vi "MQTT_TCP_Write.vi"(8 "error in (no error)":errorcluster, 9 "timeout ms (5000)":i32=5000, 10 "data in":u8[](array[numeric]) format="%x", 11 "connection ID":refnum<k5>) -> (0 "error out":errorcluster, 2 "bytes written":i32, 3 "connection ID out":refnum<k5>)   [LabVIEW 2012, in "MQTT_Functions.lvlib"]
uses:
  MQTT_Functions.lvlib
panel:
  # "this is just a wrapper for the TCP Write function\nadd or replace functionality as desired"
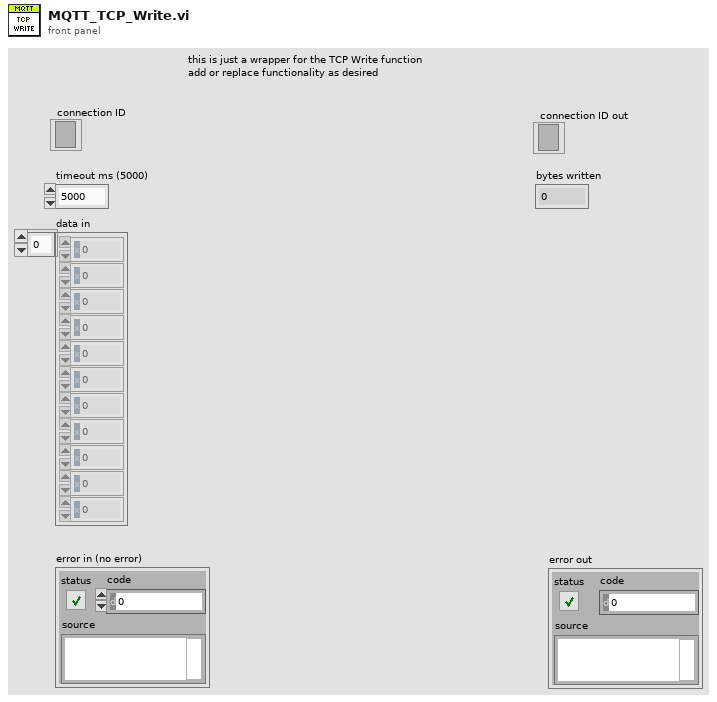
[diagram p1: front panel]
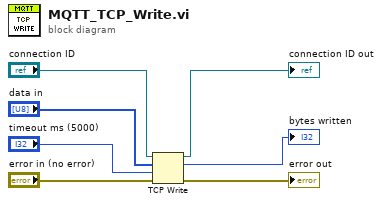
[diagram p0: block diagram]
diagram:
  n1 = TCP Write(connection ID="connection ID", data in="data in", error in (no error)="error in (no error)", 9:"timeout ms (5000)") -> (connection ID out=→"connection ID out":refnum<k5>, bytes written=→"bytes written":i32, error out=→"error out":errorcluster)
